vi "GetOutputWireBranches.vi"(6 "error in":errorcluster, 9 "CaseStructure in":refnum<class "CaseStructure.lvclass">) -> (0 "error out":errorcluster, 3 "CaseStructure out":refnum<class "CaseStructure.lvclass">, 4 "branches":string[](array[string]))   [LabVIEW 2014, in "CaseStructure.lvclass"]
uses:
  CaseStructure.lvclass
  Tunnel/Tunnel.lvclass
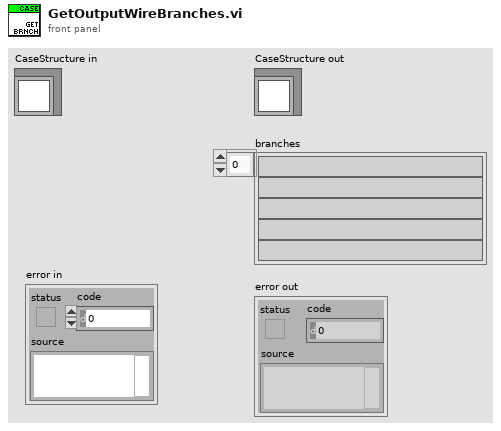
[diagram p1: front panel]
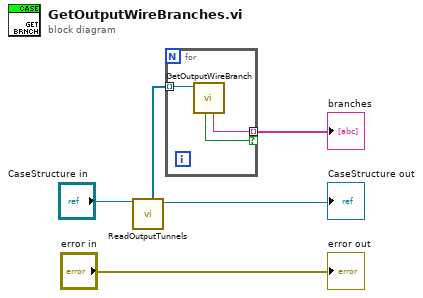
[diagram p0: block diagram]
diagram:
  n1 = call-dynamic "ReadOutputTunnels.vi"("Structure in"="CaseStructure in") -> ("Structure out"=→"CaseStructure out":refnum<class "CaseStructure.lvclass">, "outputs"=w3:refnum<class "Tunnel.lvclass">[])  [unwired: 7 in]
  n2 = for {
    tunnel: w3 -> [w8] mode=indexing
    tunnel: [w7] -> w2 mode=indexing if=w6
    n3 = call-dynamic "GetOutputWireBranch.vi"("Tunnel in"=w8) -> ("branches"=w7:string, "branched"=w6:bool)  [unwired: 5 in, 2 out]
  }
  "branches" <- w2
  "error out" <- "error in"
